vi "CAlexConfig.vi"() -> ()   [LabVIEW 2016]
uses:
  SerialChain/TypeDef/PointOnBody.ctl
  SerialChain/SerialChain.lvclass
panel:
  in  "TM-ShankCoM":T1={"Coord4"=[0.00779869, 0.00241997, 0.0611403, 1.0], "ID"=0}
  in  "TM-ShankWt":dbl=0.488 format="%#_13g"
  in  "TM-Shank-C2":T1={"Coord4"=[0.028575, -0.092075, 0.0, 1.0], "ID"=2}
  in  "TM-Shank-C1":T1={"Coord4"=[-0.104775, 0.1016, 0.0, 1.0], "ID"=1}
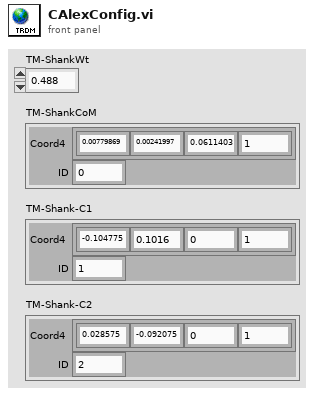
[diagram p1: front panel]
types:
  T1 = typedef "SerialChain.lvclass/PointOnBody.ctl" = cluster{"Coord4":dbl[], "ID":i32}
diagram:
